vi "Read CSM Status By CSM-VI.vi"(6 "Config Path":path, 8 "Error in":errorcluster caption="Error in (no error)", 11 "CSM VI":string) -> (0 "Error out":errorcluster, 3 "Array 3":cluster{"Status":string, "InState":string}[](array[cluster]))   [LabVIEW 2017, in "CSM-Helper API with lvcsm Support.lvlib"]
uses:
  CSM-Helper API with lvcsm Support.lvlib
  lvcsmFile/lvcsm File Support.lvlib
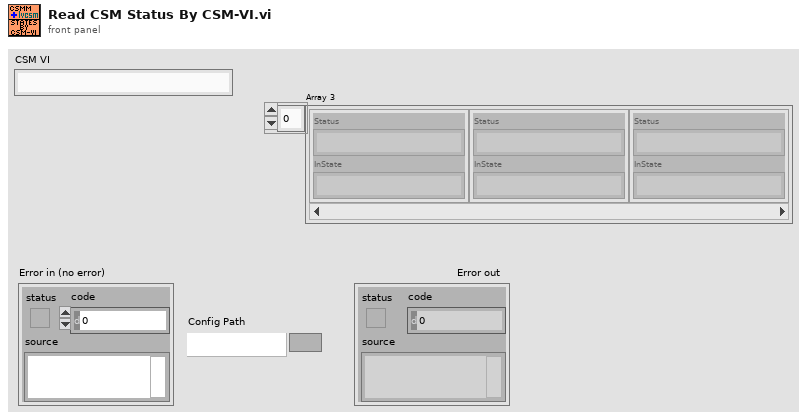
[diagram p1: front panel]
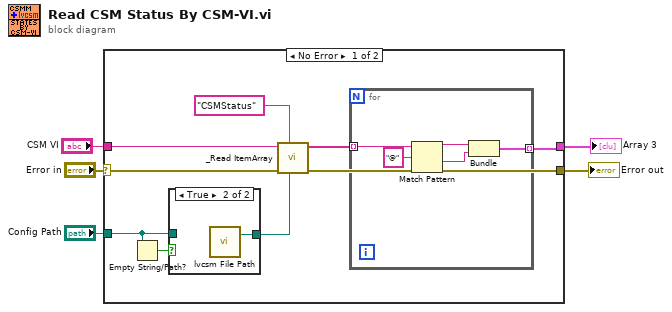
[diagram p0: block diagram]
diagram:
  n1 = case shown="No Error" "Error in" {
    selector: "Error in" -> [w12 w22]
    tunnel: [w11 w22] -> w4
    tunnel: "Config Path" -> [w14 _]
    tunnel: [w6 _] -> w2
    tunnel: "CSM VI" -> [w9 _]
    frame No Error {
      n2 = Empty String/Path?(string/path=w14) -> (empty?=w13:bool)
      n3 = case shown="True" w13 {
        tunnel: [w20 w21] -> w8
        tunnel: w14 -> [w20 _]
        frame False {
        }
        frame True {
          n4 = call "lvcsm File Path.vi"() -> ("appended path"=w21:path)  [unwired: 3 in]
        }
      }
      n5 = call "_Read ItemArray.vi"("Config Path"=w8, "Section Prefix"="CSMStatus" ("Section"), "Error in"=w12, "Section"=w9) -> ("Error out"=w11:errorcluster, "Array"=w7:string[])  [unwired: 6 in]
      n6 = for {
        tunnel: w7 -> [w19] mode=indexing
        tunnel: [w15] -> w6 mode=indexing
        n7 = Match Pattern(string=w19, regular expression="@") -> (before substring=w17:string, after substring=w16:string)  [unwired: 1 in, 2 out]
        n8 = Bundle("String"=w17, "String"=w16) -> (w15:cluster{"String":string, "String":string})  [unwired: 1 in]
      }
    }
    frame Error {
    }
  }
  "Error out" <- w4
  "Array 3" <- w2
